vi "PRO_Check Values.vi"(6 "error in (no error)":errorcluster, 7 "Full Cfg":T2={"Bench Config"={"Name"="OLR001", {"Step Levels"=0.05, "Tolerance"=0.01, "Sample Rate"=0.05, "Resistor"=100.0, "M Level Cal"=1.0, "[B Level Cal"=0.0, "Max Fill Rate"=0.025, "Empty Inches"=10.0, "Full Inches"=10.0}}, "Test Value Table "=[[98.0, 102.0, 7.91, 8.01, 7.55, 7.65, 98.0, 102.0, 7.685, 7.785, 7.325, 7.425], [197.0, 203.0, 7.46, 7.56, 7.1, 7.2, 197.0, 203.0, 7.235, 7.335, 6.875, 6.975], [296.0, 304.0, 7.01, 7.11, 6.65, 6.75, 296.0, 304.0, 6.785, 6.885, 6.425, 6.525], [395.0, 405.0, 6.56, 6.66, 6.2, 6.3, 395.0, 405.0, 6.335, 6.435, 5.975, 6.075], [494.0, 506.0, 6.11, 6.21, 5.75, 5.85, 494.0, 506.0, 5.885, 5.985, 5.525, 5.625], [593.0, 607.0, 5.66, 5.76, 5.3, 5.4, 593.0, 607.0, 5.435, 5.535, 5.075, 5.175], [692.0, 708.0, 5.21, 5.31, 4.85, 4.95, 692.0, 708.0, 4.985, 5.085, 4.625, 4.725], [791.0, 809.0, 4.76, 4.86, 4.4, 4.5, 791.0, 809.0, 4.535, 4.635, 4.175, 4.275], [890.0, 910.0, 4.31, 4.41, 3.95, 4.05, 890.0, 910.0, 4.085, 4.185, 3.725, 3.825], [989.0, 1011.0, 3.86, 3.96, 3.5, 3.6, 989.0, 1011.0, 3.635, 3.735, 3.275, 3.375], [1088.0, 1112.0, 3.41, 3.51, 3.05, 3.15, 1088.0, 1112.0, 3.185, 3.285, 2.825, 2.925]], "Table Col Titles"=[["Aohm Lo", "Aohm Hi", "A Fill Lo", "A Fill Hi", "A Drain Lo", "A Drain Hi", "Bohm Lo", "Bohm Hi", "B Fill Lo", "B Fill Hi", "B Drain Lo", "B Drain Hi"]], "Pump CtlRef In"={"Fill "=refnum, "Drain"=refnum, "Level PV"=refnum, "Flow Rate%"=refnum, "Run Test"=refnum, "Sim"=refnum, "Jog"=refnum, "Level SP"=refnum}, "Bench Status"={"Pump Status"=refnum, "Instrumnet\n Status"=refnum}}, 8 "Results in":T1=[[{"Fill"=0.0, "Drain"=7.150000000000002, "Status"=9, "Resistor"=100.0}, {"Fill"=0.0, "Drain"=6.925000000000003, "Status"=9, "Resistor"=100.0}], [{"Fill"=7.1350000000000025, "Drain"=6.700000000000004, "Status"=9, "Resistor"=200.0}, {"Fill"=6.910000000000004, "Drain"=6.475000000000005, "Status"=9, "Resistor"=200.0}], [{"Fill"=6.685000000000004, "Drain"=6.250000000000005, "Status"=9, "Resistor"=300.0}, {"Fill"=6.460000000000004, "Drain"=6.025000000000006, "Status"=9, "Resistor"=300.0}], [{"Fill"=6.235000000000006, "Drain"=5.8000000000000025, "Status"=9, "Resistor"=400.0}, {"Fill"=6.010000000000005, "Drain"=5.59, "Status"=9, "Resistor"=400.0}], [{"Fill"=5.785000000000002, "Drain"=5.364999999999997, "Status"=9, "Resistor"=500.0}, {"Fill"=5.574999999999999, "Drain"=5.1399999999999935, "Status"=9, "Resistor"=500.0}], [{"Fill"=5.349999999999996, "Drain"=4.91499999999999, "Status"=9, "Resistor"=600.0}, {"Fill"=5.124999999999993, "Drain"=4.689999999999987, "Status"=9, "Resistor"=600.0}], [{"Fill"=4.89999999999999, "Drain"=4.464999999999983, "Status"=9, "Resistor"=700.0}, {"Fill"=4.6749999999999865, "Drain"=4.23999999999998, "Status"=9, "Resistor"=700.0}], [{"Fill"=4.449999999999983, "Drain"=4.014999999999977, "Status"=9, "Resistor"=800.0}, {"Fill"=4.22499999999998, "Drain"=3.7899999999999734, "Status"=9, "Resistor"=800.0}], [{"Fill"=3.999999999999977, "Drain"=3.56499999999997, "Status"=9, "Resistor"=900.0}, {"Fill"=3.7749999999999737, "Drain"=3.339999999999967, "Status"=9, "Resistor"=900.0}], [{"Fill"=3.5499999999999705, "Drain"=3.114999999999964, "Status"=9, "Resistor"=1000.0}, {"Fill"=3.3249999999999673, "Drain"=2.8899999999999606, "Status"=9, "Resistor"=1000.0}], [{"Fill"=3.099999999999964, "Drain"=0.0, "Status"=5, "Resistor"=1100.0}, {"Fill"=2.874999999999961, "Drain"=0.0, "Status"=5, "Resistor"=1100.0}]] {"Resistor" format="%.1f"; "Drain" format="%.3f"; "Fill" format="%.3f"}, 11 "Measurement":T6=[{"Switched"=FALSE, "In Range"=TRUE, "Index"=1, "Level OUt"=8.485, " Ch n Ohms"=100.0, "Drain!Fill"=FALSE}, {"Switched"=FALSE, "In Range"=TRUE, "Index"=1, "Level OUt"=8.485, " Ch n Ohms"=100.0, "Drain!Fill"=FALSE}]) -> (0 "Results out":T1=[[{"Fill"=0.0, "Drain"=7.150000000000002, "Status"=9, "Resistor"=100.0}, {"Fill"=0.0, "Drain"=6.925000000000003, "Status"=9, "Resistor"=100.0}], [{"Fill"=7.1350000000000025, "Drain"=6.700000000000004, "Status"=9, "Resistor"=200.0}, {"Fill"=6.910000000000004, "Drain"=6.475000000000005, "Status"=9, "Resistor"=200.0}], [{"Fill"=6.685000000000004, "Drain"=6.250000000000005, "Status"=9, "Resistor"=300.0}, {"Fill"=6.460000000000004, "Drain"=6.025000000000006, "Status"=9, "Resistor"=300.0}], [{"Fill"=6.235000000000006, "Drain"=5.8000000000000025, "Status"=9, "Resistor"=400.0}, {"Fill"=6.010000000000005, "Drain"=5.59, "Status"=9, "Resistor"=400.0}], [{"Fill"=5.785000000000002, "Drain"=5.364999999999997, "Status"=9, "Resistor"=500.0}, {"Fill"=5.574999999999999, "Drain"=5.1399999999999935, "Status"=9, "Resistor"=500.0}], [{"Fill"=5.349999999999996, "Drain"=4.91499999999999, "Status"=9, "Resistor"=600.0}, {"Fill"=5.124999999999993, "Drain"=4.689999999999987, "Status"=9, "Resistor"=600.0}], [{"Fill"=4.89999999999999, "Drain"=4.464999999999983, "Status"=9, "Resistor"=700.0}, {"Fill"=4.6749999999999865, "Drain"=4.23999999999998, "Status"=9, "Resistor"=700.0}], [{"Fill"=4.449999999999983, "Drain"=4.014999999999977, "Status"=9, "Resistor"=800.0}, {"Fill"=4.22499999999998, "Drain"=3.7899999999999734, "Status"=9, "Resistor"=800.0}], [{"Fill"=3.999999999999977, "Drain"=3.56499999999997, "Status"=9, "Resistor"=900.0}, {"Fill"=3.7749999999999737, "Drain"=3.339999999999967, "Status"=9, "Resistor"=900.0}], [{"Fill"=3.5499999999999705, "Drain"=3.114999999999964, "Status"=9, "Resistor"=1000.0}, {"Fill"=3.3249999999999673, "Drain"=2.8899999999999606, "Status"=9, "Resistor"=1000.0}], [{"Fill"=3.099999999999964, "Drain"=0.0, "Status"=5, "Resistor"=1100.0}, {"Fill"=2.874999999999961, "Drain"=0.0, "Status"=5, "Resistor"=1100.0}]] {"Resistor" format="%.1f"; "Drain" format="%.3f"; "Fill" format="%.3f"}, 4 "error out":errorcluster)   [LabVIEW 2024]
uses:
  Control Definitions/Def Xresult.ctl
  Control Definitions/Def FullCfg.ctl
  Control Definitions/Def BenchCfg.ctl
  Control Definitions/Def PumpCtlRefs.ctl
  Control Definitions/Def Bench Status.ctl
  Control Definitions/Def Results2.ctl
panel:
  # "ChA=0; ChB=1"
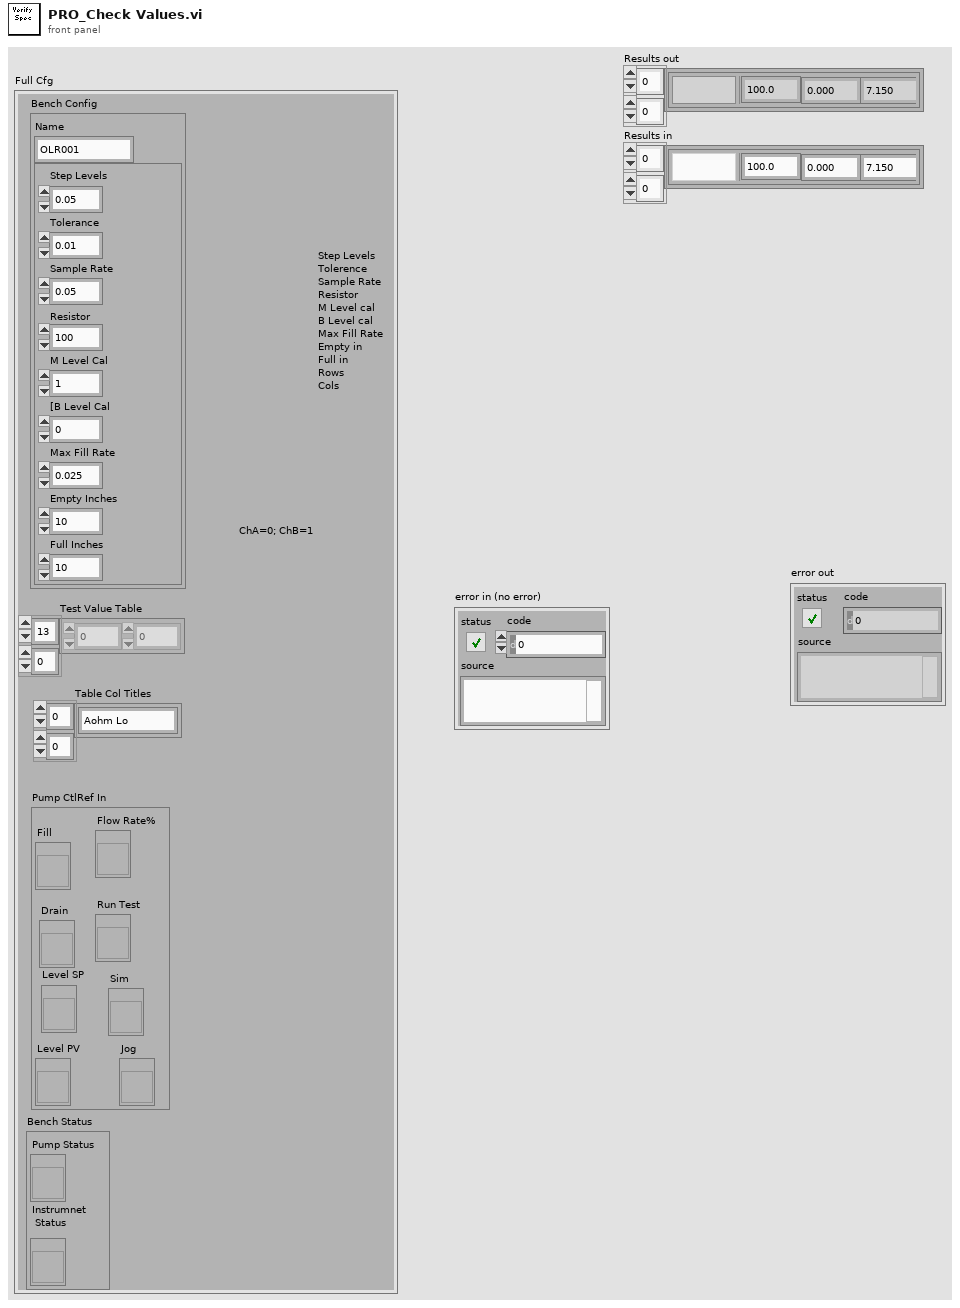
[diagram p1: front panel]
types:
  T1 = typedef "Def Results2.ctl" = cluster{"Fill":dbl, "Drain":dbl, "Status":i16, "Resistor":dbl}[][]
  T2 = typedef "Def FullCfg.ctl" = cluster{"Bench Config":T3, "Test Value Table ":dbl[][], "Table Col Titles":string[][], "Pump CtlRef In":T4, "Bench Status":T5}
  T3 = typedef "Def BenchCfg.ctl" = cluster{"Name":string, cluster{"Step Levels":dbl, "Tolerance":dbl, "Sample Rate":dbl, "Resistor":dbl, "M Level Cal":dbl, "[B Level Cal":dbl, "Max Fill Rate":dbl, "Empty Inches":dbl, "Full Inches":dbl}}
  T4 = typedef "Def PumpCtlRefs.ctl" = cluster{"Fill ":refnum<vi>, "Drain":refnum<vi>, "Level PV":refnum<vi>, "Flow Rate%":refnum<vi>, "Run Test":refnum<vi>, "Sim":refnum<vi>, "Jog":refnum<vi>, "Level SP":refnum<vi>}
  T5 = typedef "Def Bench Status.ctl" = cluster{"Pump Status":refnum<vi>, "Instrumnet\n Status":refnum<vi>}
  T6 = typedef "Def Xresult.ctl" = cluster{"Switched":bool, "In Range":bool, "Index":i16, "Level OUt":dbl, " Ch n Ohms":dbl, "Drain!Fill":bool}[]
  T7 = cluster{"Switched":bool, "In Range":bool, "Index":i16, "Level OUt":dbl, " Ch n Ohms":dbl, "Drain!Fill":bool}
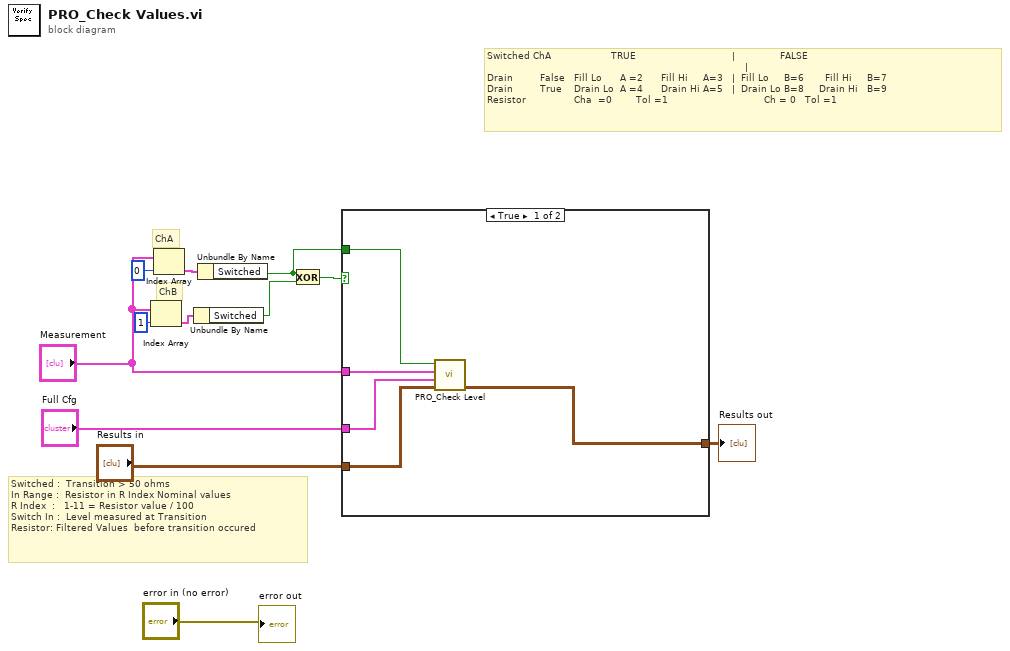
[diagram p0: block diagram]
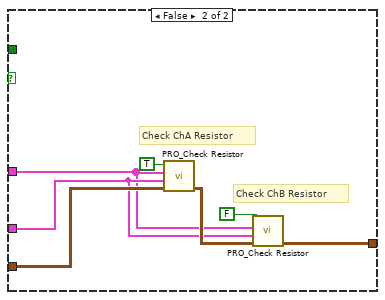
[diagram p2: hidden frame]
diagram:
  # "ChB"
  # "ChA"
  # "Switched ChA                    TRUE                                |               FALSE\n                                                                                      |\nDrain         False   Fill Lo      A =2      Fill Hi     A=3   |  Fill Lo     B=6       Fill Hi     B=7\nDrain         True    Drain Lo  A =4      Drain Hi A=5   |  Drain Lo B=8     Drain Hi   B=9 \nResistor                Cha  =0        Tol =1                                Ch = 0   Tol =1"
  # "Switched :  Transition > 50 ohms\nIn Range :  Resistor in R Index Nominal values\nR Index  :   1-11 = Resistor value / 100\nSwitch In :  Level measured at Transition\nResistor: Filtered Values  before transition occured"
  n1 = Index Array(array="Measurement", index=1) -> (element=w7:T7)
  n2 = Index Array(array="Measurement", index=0) -> (element=w8:T7)
  n3 = Unbundle By Name(w7) -> ("Switched"=w3:bool)
  n4 = Unbundle By Name(w8) -> ("Switched"=w4:bool)
  n5 = Exclusive Or(1:w3, 2:w4) -> (0:w12:bool)
  n6 = case shown="True" w12 {
    tunnel: [w13 w20] -> w2
    tunnel: "Results in" -> [w14 w24]
    tunnel: "Measurement" -> [w17 w18]
    tunnel: "Full Cfg" -> [w16 w19]
    tunnel: w4 -> [w15 _]
    frame True {
      n7 = call "PRO_Check Level.vi"("Results In in"=w14, "Full Cfg"=w16, "Measurement"=w17, "ChA/!ChB"=w15) -> ("Results In out"=w13:T1)  [unwired: 7 in]
    }
    frame False {
      # "Check ChB Resistor"
      # "Check ChA Resistor"
      n8 = call "PRO_Check Resistor.vi"("Results In in"=w24, "Full Cfg"=w19, "Measurement"=w18, "ChA/!ChB"=TRUE) -> ("Results In out"=w21:T1)  [unwired: 7 in]
      n9 = call "PRO_Check Resistor.vi"("Results In in"=w21, "Full Cfg"=w19, "Measurement"=w18, "ChA/!ChB"=FALSE) -> ("Results In out"=w20:T1)  [unwired: 7 in]
    }
  }
  "Results out" <- w2
  "error out" <- "error in (no error)"
